vi "svl_Refresh.vi"(4 "axes IN":T1 {"y axis maximum" format="%.2f"; "y axis minimum" format="%.2f"; "z axis maximum" format="%.2f"; "z axis minimum" format="%.2f"; "x axis maximum" format="%.2f"; "x axis minimum" format="%.2f"; "z axis height [%]" format="%.2f"; "x axis width [%]" format="%.2f"}, 5 "event queue IN":string[](array[string])) -> (0 "clear graph?":bool, 1 "axes OUT":T1 {"y axis maximum" format="%.2f"; "y axis minimum" format="%.2f"; "z axis maximum" format="%.2f"; "z axis minimum" format="%.2f"; "x axis maximum" format="%.2f"; "x axis minimum" format="%.2f"; "z axis height [%]" format="%.2f"; "x axis width [%]" format="%.2f"}, 2 "event queue OUT":string[](array[string]))   [LabVIEW 2017]
uses:
  <vilib>/addons/Sound and Vibration/compatibility/Waterfall/subVIs/svl_Waterfall Global.vi
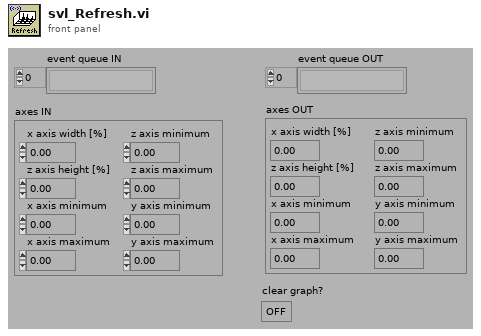
[diagram p1: front panel]
types:
  T1 = cluster{"x axis width [%]":dbl, "z axis height [%]":dbl, "x axis minimum":dbl, "x axis maximum":dbl, "z axis minimum":dbl, "z axis maximum":dbl, "y axis minimum":dbl, "y axis maximum":dbl}
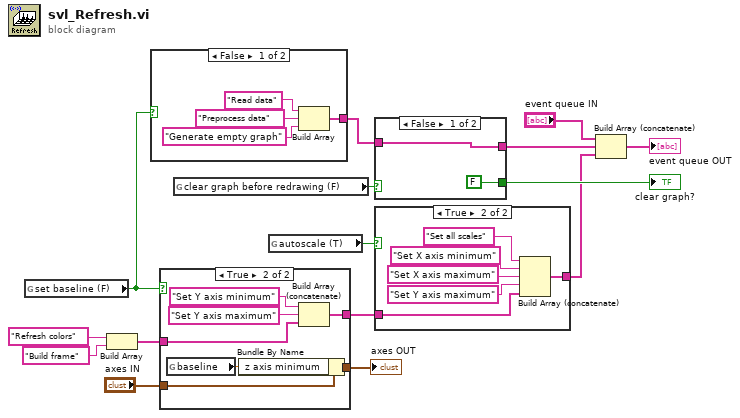
[diagram p0: block diagram]
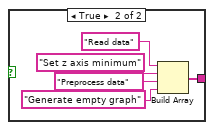
[diagram p3: hidden frame]
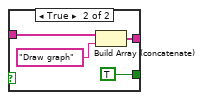
[diagram p5: hidden frame]
diagram:
  n1 = global read "svl_Waterfall Global.vi" "set baseline (F)"() -> (w8:bool)
  n2 = Build Array("Refresh colors", "Build frame") -> (w5:string[])
  n3 = case shown="False" w8 {
    tunnel: [w16 w20] -> w6
    frame False {
      n4 = Build Array("Read data", "Preprocess data", "Generate empty graph") -> (w16:string[])
    }
    frame True {
      n5 = Build Array("Read data", "Set z axis minimum", "Preprocess data", "Generate empty graph") -> (w20:string[])
    }
  }
  n6 = case shown="True" w8 {
    tunnel: w5 -> [w26 w30]
    tunnel: [w26 w31] -> w3
    tunnel: "axes IN" -> [w25 w29]
    tunnel: [w25 w27] -> w1
    frame False {
    }
    frame True {
      n7 = global read "svl_Waterfall Global.vi" "baseline"() -> (w28:dbl)
      n8 = Bundle By Name(cluster=w29, "z axis minimum"=w28) -> (w27:T1)
      n9 = Build Array (concatenate)("Set Y axis minimum", "Set Y axis maximum", w30) -> (w31:string[])
    }
  }
  "axes OUT" <- w1
  n10 = global read "svl_Waterfall Global.vi" "clear graph before redrawing (F)"() -> (w13:bool)
  n11 = global read "svl_Waterfall Global.vi" "autoscale (T)"() -> (w4:bool)
  n12 = case shown="False" w13 {
    tunnel: [FALSE TRUE] -> w12
    tunnel: w6 -> [w35 w38]
    tunnel: [w35 w36] -> w9
    frame False {
    }
    frame True {
      n13 = Build Array (concatenate)(w38, "Draw graph") -> (w36:string[])
    }
  }
  "clear graph?" <- w12
  n14 = case shown="True" w4 {
    tunnel: [w40 w41] -> w2
    tunnel: w3 -> [w40 w42]
    frame False {
    }
    frame True {
      n15 = Build Array (concatenate)("Set all scales", "Set X axis minimum", "Set X axis maximum", "Set Y axis maximum", w42) -> (w41:string[])
    }
  }
  n16 = Build Array (concatenate)("event queue IN", w9, w2) -> (→"event queue OUT":string[])
